vi "Update Armed State.vi"(8 "error in (no error)":errorcluster, 10 "Armed":bool, 11 "Pulse Recorder in":refnum<class "Pulse Recorder Actor.lvclass">) -> (0 "error out":errorcluster, 3 "Pulse Recorder out":refnum<class "Pulse Recorder Actor.lvclass">)   [LabVIEW 2021, in "Pulse Recorder Actor.lvclass"]
uses:
  Pulse Recorder Actor.lvclass
  Pulse Recorder Actor.lvclass/Pulse Recorder Actor.ctl
  Publish-Subscribe/Context.ctl
  NHMFL_Core/Libraries/Instruments/Results/Acquired Result/Acquired Result.lvclass
  Publish-Subscribe/Interfaces/Subscriber Messages/Information Msg/Information Msg.lvclass
  <vilib>/ActorFramework/Actor/Actor.lvclass
  C:/Program Files/National Instruments/LabVIEW 2021/vi.lib/ActorFramework/Actor/Actor.lvclass
  C:/GitHub/LabActor/Publish-Subscribe/Interfaces/Information/Information.lvclass
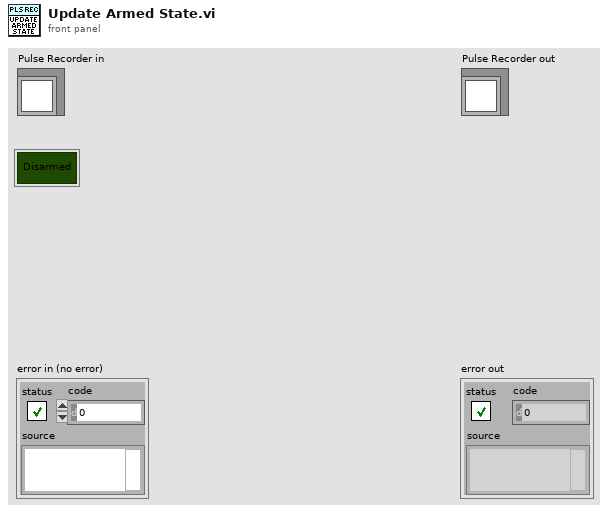
[diagram p1: front panel]
types:
  T1 = typedef "Context.ctl" = cluster{"Topic":string, "Source":string}
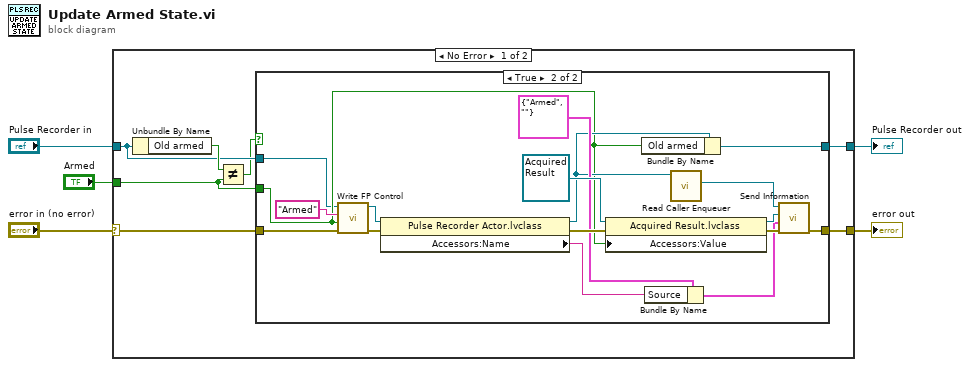
[diagram p0: block diagram]
diagram:
  n1 = case shown="No Error" "error in (no error)" {
    selector: "error in (no error)" -> [w12 w33]
    tunnel: [w11 w33] -> w4
    tunnel: [w10 w32] -> w2
    tunnel: "Pulse Recorder in" -> [w7 w32]
    tunnel: "Armed" -> [w8 _]
    frame No Error {
      n2 = Unbundle By Name(w7) -> ("Old armed"=w9:bool)
      n3 = Not Equal?(x=w9, y=w8) -> (x != y?=w6:bool)
      n4 = case shown="True" w6 {
        tunnel: w12 -> [w13 w26]
        tunnel: [w13 w19] -> w11
        tunnel: [w14 w17] -> w10
        tunnel: w8 -> [_ w16]
        tunnel: w7 -> [w14 w15]
        frame False {
        }
        frame True {
          n5 = call-dynamic "Write FP Control.vi"("error in (no error)"=w26, "Control Value"=w16, "Control Name"="Armed", "Measure Object in"=w15) -> ("error out"=w27:errorcluster, "Measure Object out"=w28:refnum<class "Pulse Recorder Actor.lvclass">)  [unwired: 6 in]
          n6 = property class="Pulse Recorder Actor.lvclass"(reference=w28, error in=w27) -> (reference out=w18:refnum<class "Pulse Recorder Actor.lvclass">, error out=w30:errorcluster, "Accessors:Name"=w31:string)
          n7 = property class="Acquired Result.lvclass"(reference=refnum<class "Acquired Result.lvclass"> refnum ("Acquired Result.lvclass"), error in=w30, "Accessors:Value"=w16) -> (reference out=w25:refnum<class "Acquired Result.lvclass">, error out=w24:errorcluster)
          n8 = Bundle By Name(cluster=w18, "Old armed"=w16) -> (w17:refnum<class "Pulse Recorder Actor.lvclass">)
          n9 = Bundle By Name(cluster=T1 {"Topic"="Armed", "Source"=""} ("Context"), "Source"=w31) -> (w23:T1)
          n10 = call <vilib>:"Read Caller Enqueuer.vi"("Actor"=w18) -> ("Caller Enqueuer"=w22:refnum<class "Message Enqueuer.lvclass">)  [unwired: 10 in]
          n11 = call "Send Information.vi"("error in (no error)"=w24, "Context"=w23, "Information"=w25, "Message Enqueuer"=w22) -> ("error out"=w19:errorcluster)  [unwired: 6 in, 1 out]
        }
      }
    }
    frame Error {
    }
  }
  "error out" <- w4
  "Pulse Recorder out" <- w2
